vi "Result.Numeric, Compare Value to Limits.vi"(8 "UL":dbl, 9 "LL":dbl, 10 "Value":dbl, 11 "LimType":T2) -> (3 "Status":T1=3 items=["LOG", "PASS", "FAIL", "ERROR"])   [LabVIEW 2018]
uses:
  Result.Limit Type.ctl
  Result.Measurement and Attribute Item Status.ctl
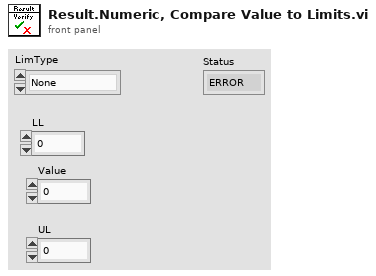
[diagram p1: front panel]
types:
  T1 = typedef "Result.Measurement and Attribute Item Status.ctl" = i32
  T2 = typedef "Result.Limit Type.ctl" = enum16{"None", "EQ", "NE", "GT", "LT", "GE", "LE", "GTLT", "GELE", "GELT", "GTLE", "LTGT", "LEGE", "LEGT", "LTGE", "Contains", "NotContains"}
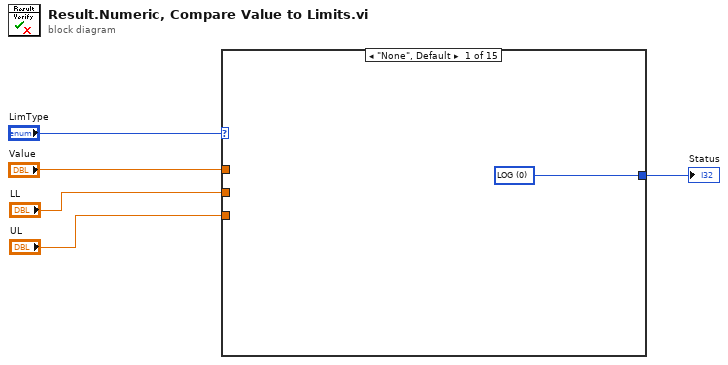
[diagram p0: block diagram]
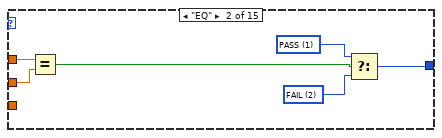
[diagram p2: hidden frame]
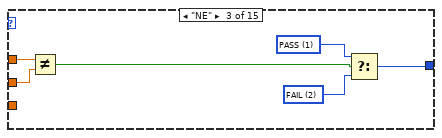
[diagram p3: hidden frame]
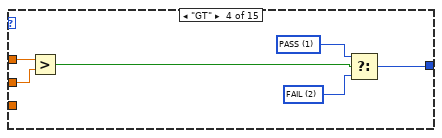
[diagram p4: hidden frame]
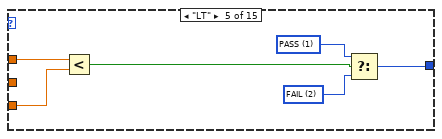
[diagram p5: hidden frame]
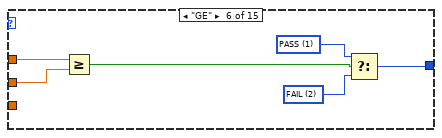
[diagram p6: hidden frame]
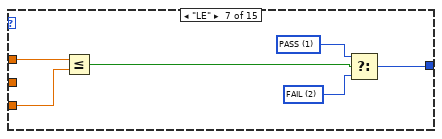
[diagram p7: hidden frame]
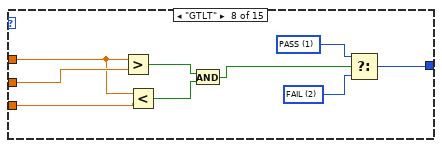
[diagram p8: hidden frame]
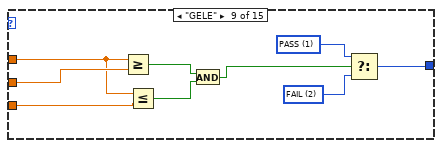
[diagram p9: hidden frame]
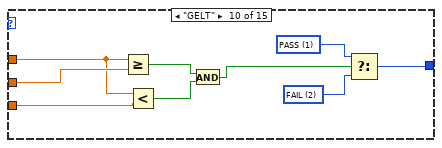
[diagram p10: hidden frame]
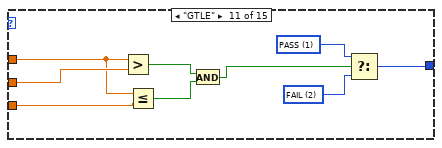
[diagram p11: hidden frame]
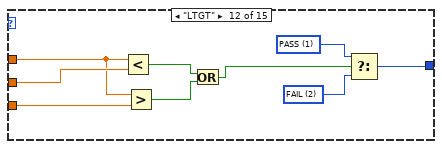
[diagram p12: hidden frame]
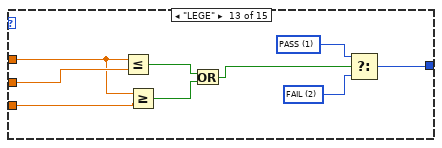
[diagram p13: hidden frame]
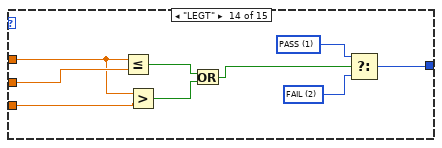
[diagram p14: hidden frame]
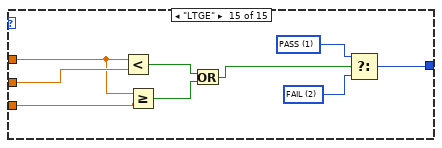
[diagram p15: hidden frame]
diagram:
  n1 = case shown="\"None\", Default" "LimType" {
    tunnel: "Value" -> [_ w12 w18 w24 w30 w32 w38 w47 w56 w65 w74 w83 w92 w101 w110]
    tunnel: "LL" -> [_ w11 w17 w23 _ w31 _ w48 w57 w66 w75 w84 w93 w102 w111]
    tunnel: "UL" -> [_ _ _ _ w25 _ w37 w46 w55 w64 w73 w82 w91 w100 w109]
    tunnel: [w6 w10 w16 w22 w29 w36 w42 w51 w60 w69 w78 w87 w96 w105 w114] -> w1
    frame "None", Default {
      w6 = T1 0 items=["LOG", "PASS", "FAIL", "ERROR"] ("Status")
    }
    frame "EQ" {
      w8 = T1 2 items=["LOG", "PASS", "FAIL", "ERROR"] ("Status")
      w9 = T1 1 items=["LOG", "PASS", "FAIL", "ERROR"] ("Status")
      n2 = Equal?(x=w12, y=w11) -> (x = y?=w7:bool)
      n3 = Select(t=w9, s=w7, f=w8) -> (s? t:f=w10:T1)
    }
    frame "NE" {
      w14 = T1 2 items=["LOG", "PASS", "FAIL", "ERROR"] ("Status")
      w15 = T1 1 items=["LOG", "PASS", "FAIL", "ERROR"] ("Status")
      n4 = Not Equal?(x=w18, y=w17) -> (x != y?=w13:bool)
      n5 = Select(t=w15, s=w13, f=w14) -> (s? t:f=w16:T1)
    }
    frame "GT" {
      w20 = T1 2 items=["LOG", "PASS", "FAIL", "ERROR"] ("Status")
      w21 = T1 1 items=["LOG", "PASS", "FAIL", "ERROR"] ("Status")
      n6 = Greater?(x=w24, y=w23) -> (0:w19:bool)
      n7 = Select(t=w21, s=w19, f=w20) -> (s? t:f=w22:T1)
    }
    frame "LT" {
      w27 = T1 2 items=["LOG", "PASS", "FAIL", "ERROR"] ("Status")
      w28 = T1 1 items=["LOG", "PASS", "FAIL", "ERROR"] ("Status")
      n8 = Less?(x=w30, y=w25) -> (x < y?=w26:bool)
      n9 = Select(t=w28, s=w26, f=w27) -> (s? t:f=w29:T1)
    }
    frame "GE" {
      w34 = T1 2 items=["LOG", "PASS", "FAIL", "ERROR"] ("Status")
      w35 = T1 1 items=["LOG", "PASS", "FAIL", "ERROR"] ("Status")
      n10 = Greater Or Equal?(x=w32, y=w31) -> (x >= y?=w33:bool)
      n11 = Select(t=w35, s=w33, f=w34) -> (s? t:f=w36:T1)
    }
    frame "LE" {
      w40 = T1 2 items=["LOG", "PASS", "FAIL", "ERROR"] ("Status")
      w41 = T1 1 items=["LOG", "PASS", "FAIL", "ERROR"] ("Status")
      n12 = Less Or Equal?(x=w38, y=w37) -> (x <= y?=w39:bool)
      n13 = Select(t=w41, s=w39, f=w40) -> (s? t:f=w42:T1)
    }
    frame "GTLT" {
      w49 = T1 2 items=["LOG", "PASS", "FAIL", "ERROR"] ("Status")
      w50 = T1 1 items=["LOG", "PASS", "FAIL", "ERROR"] ("Status")
      n14 = Greater?(x=w47, y=w48) -> (0:w45:bool)
      n15 = Less?(x=w47, y=w46) -> (x < y?=w44:bool)
      n16 = And(x=w45, y=w44) -> (x .and. y?=w43:bool)
      n17 = Select(t=w50, s=w43, f=w49) -> (s? t:f=w51:T1)
    }
    frame "GELE" {
      w58 = T1 2 items=["LOG", "PASS", "FAIL", "ERROR"] ("Status")
      w59 = T1 1 items=["LOG", "PASS", "FAIL", "ERROR"] ("Status")
      n18 = Greater Or Equal?(x=w56, y=w57) -> (x >= y?=w54:bool)
      n19 = Less Or Equal?(x=w56, y=w55) -> (x <= y?=w53:bool)
      n20 = And(x=w54, y=w53) -> (x .and. y?=w52:bool)
      n21 = Select(t=w59, s=w52, f=w58) -> (s? t:f=w60:T1)
    }
    frame "GELT" {
      w67 = T1 2 items=["LOG", "PASS", "FAIL", "ERROR"] ("Status")
      w68 = T1 1 items=["LOG", "PASS", "FAIL", "ERROR"] ("Status")
      n22 = Greater Or Equal?(x=w65, y=w66) -> (x >= y?=w63:bool)
      n23 = Less?(x=w65, y=w64) -> (x < y?=w62:bool)
      n24 = And(x=w63, y=w62) -> (x .and. y?=w61:bool)
      n25 = Select(t=w68, s=w61, f=w67) -> (s? t:f=w69:T1)
    }
    frame "GTLE" {
      w76 = T1 2 items=["LOG", "PASS", "FAIL", "ERROR"] ("Status")
      w77 = T1 1 items=["LOG", "PASS", "FAIL", "ERROR"] ("Status")
      n26 = Greater?(x=w74, y=w75) -> (0:w72:bool)
      n27 = Less Or Equal?(x=w74, y=w73) -> (x <= y?=w71:bool)
      n28 = And(x=w72, y=w71) -> (x .and. y?=w70:bool)
      n29 = Select(t=w77, s=w70, f=w76) -> (s? t:f=w78:T1)
    }
    frame "LTGT" {
      w85 = T1 2 items=["LOG", "PASS", "FAIL", "ERROR"] ("Status")
      w86 = T1 1 items=["LOG", "PASS", "FAIL", "ERROR"] ("Status")
      n30 = Less?(x=w83, y=w84) -> (x < y?=w81:bool)
      n31 = Greater?(x=w83, y=w82) -> (0:w80:bool)
      n32 = Or(x=w81, y=w80) -> (x .or. y?=w79:bool)
      n33 = Select(t=w86, s=w79, f=w85) -> (s? t:f=w87:T1)
    }
    frame "LEGE" {
      w94 = T1 2 items=["LOG", "PASS", "FAIL", "ERROR"] ("Status")
      w95 = T1 1 items=["LOG", "PASS", "FAIL", "ERROR"] ("Status")
      n34 = Less Or Equal?(x=w92, y=w93) -> (x <= y?=w90:bool)
      n35 = Greater Or Equal?(x=w92, y=w91) -> (x >= y?=w89:bool)
      n36 = Or(x=w90, y=w89) -> (x .or. y?=w88:bool)
      n37 = Select(t=w95, s=w88, f=w94) -> (s? t:f=w96:T1)
    }
    frame "LEGT" {
      w103 = T1 2 items=["LOG", "PASS", "FAIL", "ERROR"] ("Status")
      w104 = T1 1 items=["LOG", "PASS", "FAIL", "ERROR"] ("Status")
      n38 = Less Or Equal?(x=w101, y=w102) -> (x <= y?=w99:bool)
      n39 = Greater?(x=w101, y=w100) -> (0:w98:bool)
      n40 = Or(x=w99, y=w98) -> (x .or. y?=w97:bool)
      n41 = Select(t=w104, s=w97, f=w103) -> (s? t:f=w105:T1)
    }
    frame "LTGE" {
      w112 = T1 2 items=["LOG", "PASS", "FAIL", "ERROR"] ("Status")
      w113 = T1 1 items=["LOG", "PASS", "FAIL", "ERROR"] ("Status")
      n42 = Less?(x=w110, y=w111) -> (x < y?=w108:bool)
      n43 = Greater Or Equal?(x=w110, y=w109) -> (x >= y?=w107:bool)
      n44 = Or(x=w108, y=w107) -> (x .or. y?=w106:bool)
      n45 = Select(t=w113, s=w106, f=w112) -> (s? t:f=w114:T1)
    }
  }
  "Status" <- w1
